vi "Read Configuration.vi"(8 "error in (no error)":errorcluster, 11 "Lotis in":refnum<class "PL Lotis TII LS.lvclass">) -> (0 "error out":errorcluster, 2 "configuration":T1={"device mode"=0, "error code"=0, "number of errors"=0, "cooling system"={"ready"=FALSE, "error"=FALSE}, "lamps"={"frequency, Hz"=0, "channel 1"={"trigger"=1, "state"=1, "energy, J"=0.0}, "channel 2"={"trigger"=1, "state"=1, "energy, J"=0.0}, "amplifier"={"enabled"=FALSE}, "off delay, s"=0, "number of shots"=0, "operation time, min."=0}, "Q-switches"={"frequency, Hz"=0.0, "trigger"=1, "channel 1"={"on"=FALSE, "delay, ns"=0}, "channel 2"={"on"=FALSE, "delay ,ns"=0}, "number of shots"=0}, "shutters"={"channel 1"={"open"=FALSE}, "channel 2"={"open"=FALSE}}, "external device state index"=0, "exernal device flags"=[], "radiation energy, mJ"={"channel 1"=0, "channel 2"=0}, "lamp to Q-switch frequency ratio"=0, "4th harmonic crystal T, °C"=0.0} {"Q-switches"."trigger" items=["always on", "internal", "external (primary)", "external (secondary)", "single shot"]; "device mode" items=["independent", "primary", "secondary"]; "lamps"."channel 2"."state" items=["off"=0, "on"=1, "pulses"=3]; "lamps"."channel 2"."trigger" items=["internal"=1, "external"=2, "single shot"=3]; "lamps"."channel 1"."state" items=["off"=0, "on"=1, "pulses"=3]; "lamps"."channel 1"."trigger" items=["internal"=1, "external"=2, "single shot"=3]}, 3 "Lotis out":refnum<class "PL Lotis TII LS.lvclass">)   [LabVIEW 2015, in "PL Lotis TII LS.lvclass"]
doc: "Reads device configuration and state."
uses:
  PL Lotis TII LS.lvclass
panel:
  out "response 2":string
  out "response 1":string
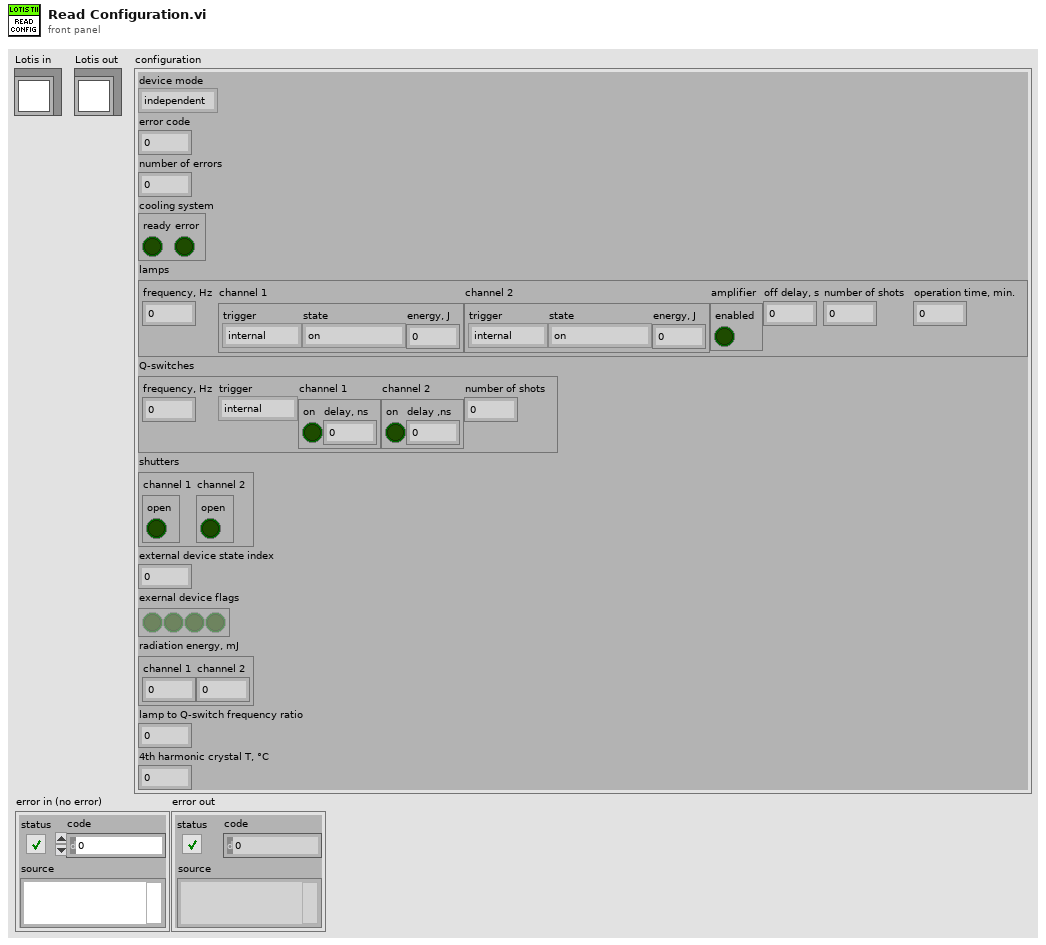
[diagram p1: front panel]
types:
  T1 = cluster{"device mode":u16, "error code":u8, "number of errors":u8, "cooling system":cluster{"ready":bool, "error":bool}, "lamps":cluster{"frequency, Hz":u32, "channel 1":cluster{"trigger":u16, "state":u16, "energy, J":dbl}, "channel 2":cluster{"trigger":u16, "state":u16, "energy, J":dbl}, "amplifier":cluster{"enabled":bool}, "off delay, s":u32, "number of shots":u32, "operation time, min.":u32}, "Q-switches":cluster{"frequency, Hz":dbl, "trigger":u16, "channel 1":cluster{"on":bool, "delay, ns":u32}, "channel 2":cluster{"on":bool, "delay ,ns":u32}, "number of shots":u32}, "shutters":cluster{"channel 1":cluster{"open":bool}, "channel 2":cluster{"open":bool}}, "external device state index":u8, "exernal device flags":bool[], "radiation energy, mJ":cluster{"channel 1":u32, "channel 2":u32}, "lamp to Q-switch frequency ratio":u32, "4th harmonic crystal T, °C":dbl}
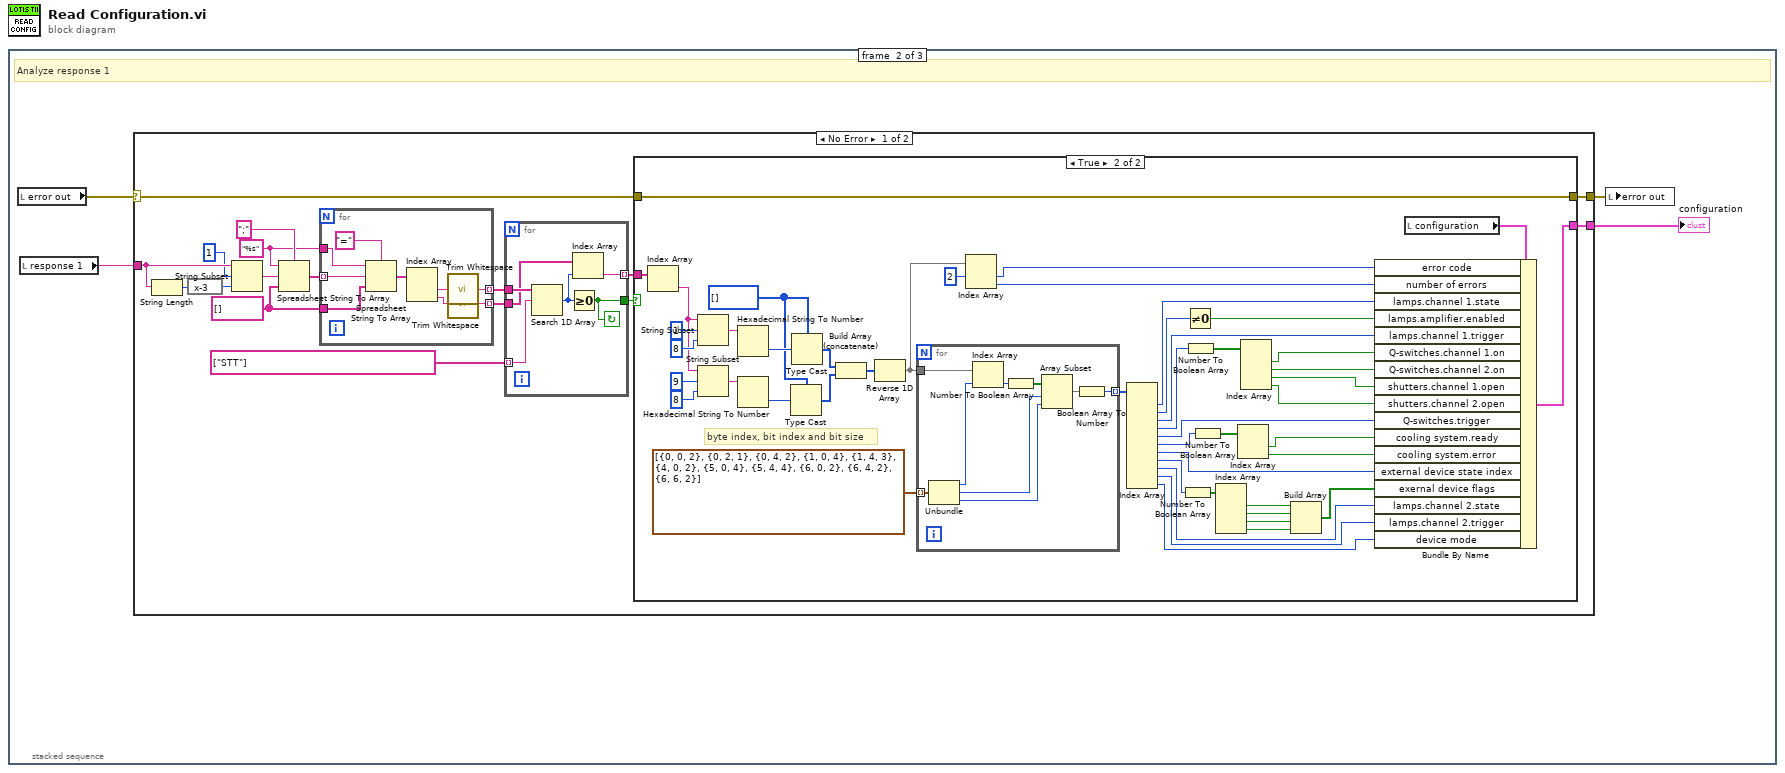
[diagram p0: block diagram]
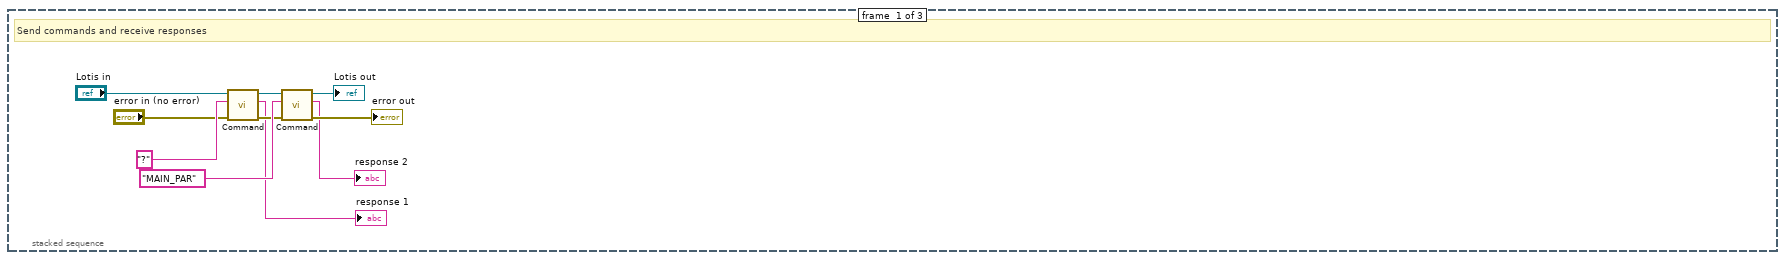
[diagram p2: hidden frame]
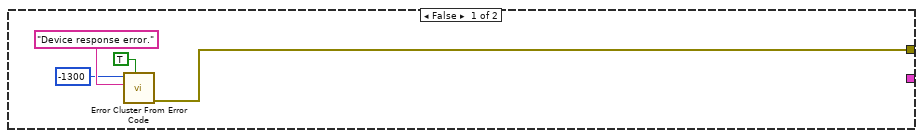
[diagram p3: hidden frame]
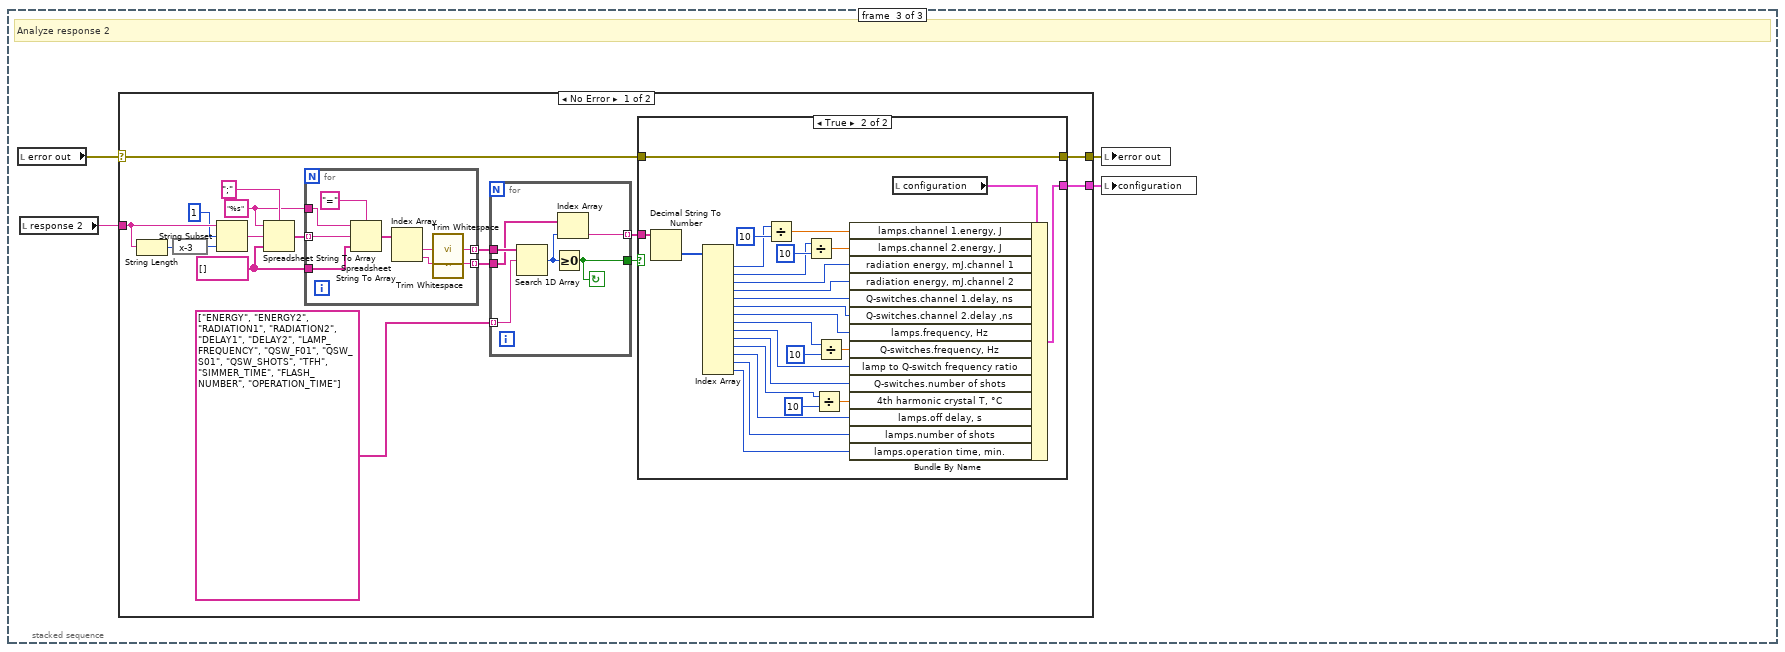
[diagram p5: hidden frame]
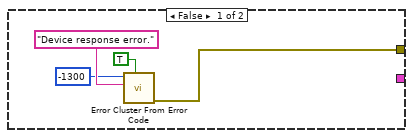
[diagram p6: hidden frame]
diagram:
  n1 = stacked-sequence {
    frame #0 {
      # "Send commands and receive responses"
      n2 = call "Command.vi"("error in (no error)"="error in (no error)", "command"="?", "Lotis in"="Lotis in") -> ("error out"=w7:errorcluster, "response data"=→"response 1":string, "Lotis out"=w6:refnum<class "PL Lotis TII LS.lvclass">)  [unwired: 6 in]
      n3 = call "Command.vi"("error in (no error)"=w7, "command"="MAIN_PAR", "Lotis in"=w6) -> ("error out"=→"error out":errorcluster, "response data"=→"response 2":string, "Lotis out"=→"Lotis out":refnum<class "PL Lotis TII LS.lvclass">)  [unwired: 6 in]
    }
    frame #1 {
      # "Analyze response 1"
      n4 = local read "error out"() -> (w14:errorcluster)
      n5 = local read "response 1"() -> (w11:string)
      n6 = case shown="No Error" w14 {
        selector: w14 -> [w20 w109]
        tunnel: w11 -> [w31 _]
        tunnel: [w19 w109] -> w13
        tunnel: [w15 _] -> w12
        frame No Error {
          w24 = "%s" ("format string")
          w23 = string[] [] ("array type (2D Dbl)")
          n7 = String Length(string=w31) -> (length=w29:i32)
          n8 = expression code="x-3"(w29) -> (w28:i32)
          n9 = String Subset(string=w31, offset (0)=1, length (rest)=w28) -> (substring=w27:string)
          n10 = Spreadsheet String To Array(delimiter (Tab)=";", format string=w24, spreadsheet string=w27, array type (2D Dbl)=w23) -> (array=w25:string[])
          n11 = for {
            tunnel: w25 -> [w105] mode=indexing
            tunnel: w24 -> [w108]
            tunnel: w23 -> [w106]
            tunnel: [w101] -> w22 mode=indexing
            tunnel: [w100] -> w17 mode=indexing
            n12 = Spreadsheet String To Array(delimiter (Tab)="=", format string=w108, spreadsheet string=w105, array type (2D Dbl)=w106) -> (array=w104:string[])
            n13 = Index Array(array=w104) -> (element #1=w103:string, element #2=w102:string)  [unwired: 2 in]
            n14 = call <vilib>:"Trim Whitespace.vi"("string"=w103) -> ("trimmed string"=w101:string)  [unwired: 1 in]
            n15 = call <vilib>:"Trim Whitespace.vi"("string"=w102) -> ("trimmed string"=w100:string)  [unwired: 1 in]
          }
          n16 = for {
            tunnel: w22 -> [w99]
            tunnel: string[] ["STT"] -> [w98] mode=indexing
            tunnel: [w97] -> w18
            tunnel: w17 -> [w96]
            tunnel: [w94] -> w16 mode=indexing
            stop <- w97 continue-if-true
            n17 = Search 1D Array(1D array=w99, element=w98) -> (index of element=w95:i32)  [unwired: 1 in]
            n18 = Greater Or Equal To 0?(x=w95) -> (x >= 0?=w97:bool)
            n19 = Index Array(array=w96, index=w95) -> (element=w94:string)
          }
          n20 = case shown="True" w18 {
            tunnel: w20 -> [_ w84]
            tunnel: [w32 w84] -> w19
            tunnel: w16 -> [_ w81]
            tunnel: [_ w82] -> w15
            frame False {
              n21 = call <vilib>:"Error Cluster From Error Code.vi"("show call chain? (False)"=TRUE, "error message (\"\")"="Device response error." ("format string"), "error code (0)"=-1300) -> ("error out"=w32:errorcluster)  [unwired: 6 in]
            }
            frame True {
              w72 = u8[] []
              # "byte index, bit index and bit size"
              n22 = Index Array(array=w81) -> (element=w66:string)  [unwired: 1 in]
              n23 = String Subset(string=w66, offset (0)=1, length (rest)=8 ("length (rest)")) -> (substring=w76:string)
              n24 = String Subset(string=w66, offset (0)=9, length (rest)=8 ("length (rest)")) -> (substring=w75:string)
              n25 = Hexadecimal String To Number(string=w76) -> (number=w74:u32)  [unwired: 2 in, 1 out]
              n26 = Hexadecimal String To Number(string=w75) -> (number=w73:u32)  [unwired: 2 in, 1 out]
              n27 = Type Cast(type=w72, x=w73) -> (*(type *) &x=w70:u8[])
              n28 = Type Cast(type=w72, x=w74) -> (*(type *) &x=w71:u8[])
              n29 = Build Array (concatenate)(w71, w70) -> (w69:u8[])
              n30 = Reverse 1D Array(array=w69) -> (reversed array=w65:u8[])
              n31 = for {
                tunnel: w65 -> [w93]
                tunnel: cluster{i32, i32, i32}[] [{0, 0, 2}, {0, 2, 1}, {0, 4, 2}, {1, 0, 4}, {1, 4, 3}, {4, 0, 2}, {5, 0, 4}, {5, 4, 4}, {6, 0, 2}, {6, 4, 2}, {6, 6, 2}] -> [w92] mode=indexing
                tunnel: [w85] -> w67 mode=indexing
                n32 = Unbundle(w92) -> (w91:i32, w88:i32, w87:i32)
                n33 = Index Array(array=w93, index=w91) -> (element=w90:u8)
                n34 = Number To Boolean Array(number=w90) -> (Boolean array=w89:bool[])
                n35 = Array Subset(array=w89, index=w88, length=w87) -> (w86:bool[])
                n36 = Boolean Array To Number(Boolean array=w86) -> (number=w85:u32)
              }
              n37 = Index Array(array=w65, index #1=2 ("index")) -> (element #1=w63:u8, element #2=w62:u8)  [unwired: 1 in]
              n38 = Index Array(array=w67) -> (element #1=w61:u32, element #2=w60:u32, element #3=w58:u32, element #4=w55:u32, element #5=w49:u32, element #6=w48:u32, element #7=w44:u32, element #8=w43:u32, element #9=w42:u32, element #10=w41:u32, element #11=w40:u32)  [unwired: 11 in]
              n39 = Number To Boolean Array(number=w43) -> (Boolean array=w57:bool[])
              n40 = Not Equal To 0?(x=w60) -> (x != 0?=w59:bool)
              n41 = Number To Boolean Array(number=w55) -> (Boolean array=w54:bool[])
              n42 = Number To Boolean Array(number=w48) -> (Boolean array=w47:bool[])
              n43 = Index Array(array=w57) -> (element #1=w39:bool, element #2=w38:bool, element #3=w37:bool, element #4=w36:bool)  [unwired: 4 in]
              n44 = Index Array(array=w47) -> (element #1=w46:bool, element #2=w45:bool)  [unwired: 2 in]
              n45 = Index Array(array=w54) -> (element #1=w53:bool, element #2=w52:bool, element #3=w50:bool, element #4=w51:bool)  [unwired: 4 in]
              n46 = Build Array(w39, w38, w37, w36) -> (w56:bool[])
              n47 = local read "configuration"() -> (w83:T1)
              n48 = Bundle By Name(cluster=w83, "error code"=w63, "number of errors"=w62, "lamps.channel 1.state"=w61, "lamps.amplifier.enabled"=w59, "lamps.channel 1.trigger"=w58, "Q-switches.channel 1.on"=w53, "Q-switches.channel 2.on"=w52, "shutters.channel 1.open"=w50, "shutters.channel 2.open"=w51, "Q-switches.trigger"=w49, "cooling system.ready"=w46, "cooling system.error"=w45, "external device state index"=w44, "exernal device flags"=w56, "lamps.channel 2.state"=w42, "lamps.channel 2.trigger"=w41, "device mode"=w40) -> (w82:T1)
            }
          }
        }
        frame Error {
        }
      }
      "configuration" <- w12
      n49 = local write "error out"(w13) -> ()
    }
    frame #2 {
      # "Analyze response 2"
      n50 = local read "error out"() -> (w113:errorcluster)
      n51 = local read "response 2"() -> (w111:string)
      n52 = case shown="No Error" w113 {
        selector: w113 -> [w119 w177]
        tunnel: w111 -> [w130 _]
        tunnel: [w118 w177] -> w112
        tunnel: [w114 _] -> w110
        frame No Error {
          w123 = "%s" ("format string")
          w122 = string[] [] ("array type (2D Dbl)")
          n53 = String Length(string=w130) -> (length=w128:i32)
          n54 = expression code="x-3"(w128) -> (w127:i32)
          n55 = String Subset(string=w130, offset (0)=1, length (rest)=w127) -> (substring=w126:string)
          n56 = Spreadsheet String To Array(delimiter (Tab)=";", format string=w123, spreadsheet string=w126, array type (2D Dbl)=w122) -> (array=w124:string[])
          n57 = for {
            tunnel: w124 -> [w173] mode=indexing
            tunnel: w123 -> [w176]
            tunnel: w122 -> [w174]
            tunnel: [w169] -> w121 mode=indexing
            tunnel: [w168] -> w116 mode=indexing
            n58 = Spreadsheet String To Array(delimiter (Tab)="=", format string=w176, spreadsheet string=w173, array type (2D Dbl)=w174) -> (array=w172:string[])
            n59 = Index Array(array=w172) -> (element #1=w171:string, element #2=w170:string)  [unwired: 2 in]
            n60 = call <vilib>:"Trim Whitespace.vi"("string"=w171) -> ("trimmed string"=w169:string)  [unwired: 1 in]
            n61 = call <vilib>:"Trim Whitespace.vi"("string"=w170) -> ("trimmed string"=w168:string)  [unwired: 1 in]
          }
          n62 = for {
            tunnel: w121 -> [w167]
            tunnel: string[] ["ENERGY", "ENERGY2", "RADIATION1", "RADIATION2", "DELAY1", "DELAY2", "LAMP_FREQUENCY", "QSW_F01", "QSW_S01", "QSW_SHOTS", "TFH", "SIMMER_TIME", "FLASH_NUMBER", "OPERATION_TIME"] -> [w166] mode=indexing
            tunnel: [w165] -> w117
            tunnel: w116 -> [w164]
            tunnel: [w162] -> w115 mode=indexing
            stop <- w165 continue-if-true
            n63 = Search 1D Array(1D array=w167, element=w166) -> (index of element=w163:i32)  [unwired: 1 in]
            n64 = Greater Or Equal To 0?(x=w163) -> (x >= 0?=w165:bool)
            n65 = Index Array(array=w164, index=w163) -> (element=w162:string)
          }
          n66 = case shown="True" w117 {
            tunnel: w119 -> [_ w161]
            tunnel: [w131 w161] -> w118
            tunnel: w115 -> [_ w158]
            tunnel: [_ w159] -> w114
            frame False {
              n67 = call <vilib>:"Error Cluster From Error Code.vi"("show call chain? (False)"=TRUE, "error message (\"\")"="Device response error." ("format string"), "error code (0)"=-1300) -> ("error out"=w131:errorcluster)  [unwired: 6 in]
            }
            frame True {
              n68 = Decimal String To Number(string=w158) -> (number=w157:i32[])  [unwired: 2 in, 1 out]
              n69 = Index Array(array=w157) -> (element #1=w141:i32, element #2=w138:i32, element #3=w156:i32, element #4=w155:i32, element #5=w154:i32, element #6=w153:i32, element #7=w152:i32, element #8=w151:i32, element #9=w148:i32, element #10=w147:i32, element #11=w135:i32, element #12=w146:i32, element #13=w145:i32, element #14=w144:i32)  [unwired: 14 in]
              n70 = Divide(x=w141, y=10) -> (x/y=w142:dbl)
              n71 = Divide(x=w138, y=10) -> (x/y=w139:dbl)
              n72 = Divide(x=w135, y=10) -> (x/y=w136:dbl)
              n73 = Divide(x=w151, y=10) -> (x/y=w150:dbl)
              n74 = local read "configuration"() -> (w160:T1)
              n75 = Bundle By Name(cluster=w160, "lamps.channel 1.energy, J"=w142, "lamps.channel 2.energy, J"=w139, "radiation energy, mJ.channel 1"=w156, "radiation energy, mJ.channel 2"=w155, "Q-switches.channel 1.delay, ns"=w154, "Q-switches.channel 2.delay ,ns"=w153, "lamps.frequency, Hz"=w152, "Q-switches.frequency, Hz"=w150, "lamp to Q-switch frequency ratio"=w148, "Q-switches.number of shots"=w147, "4th harmonic crystal T, °C"=w136, "lamps.off delay, s"=w146, "lamps.number of shots"=w145, "lamps.operation time, min."=w144) -> (w159:T1)
            }
          }
        }
        frame Error {
        }
      }
      n76 = local write "error out"(w112) -> ()
      n77 = local write "configuration"(w110) -> ()
    }
  }
